vi "Get ICM Setting.vi"(8 "error in (no error)":errorcluster, 10 "Scan Data Process in":T1, 11 "tdms file":refnum<k34>) -> (0 "error out":errorcluster, 2 "Scan Data Process out":T1, 3 "tdms file out":refnum<k34>, 4 "Vaild?":bool)   [LabVIEW 2015, in "Exposure Process.lvlib"]
uses:
  Exposure Process.lvlib
  Control_Scan Data Process.ctl
  <vilib>/addons/PointValueMap/controls/PointMap.ctl
  Control_EXP Information.ctl
  Control_File Save Setup.ctl
  Control_Enable and Path.ctl
  Control_ICM Export Setting.ctl
  <vilib>/addons/PointValueMap/PointValueMap.lvlib
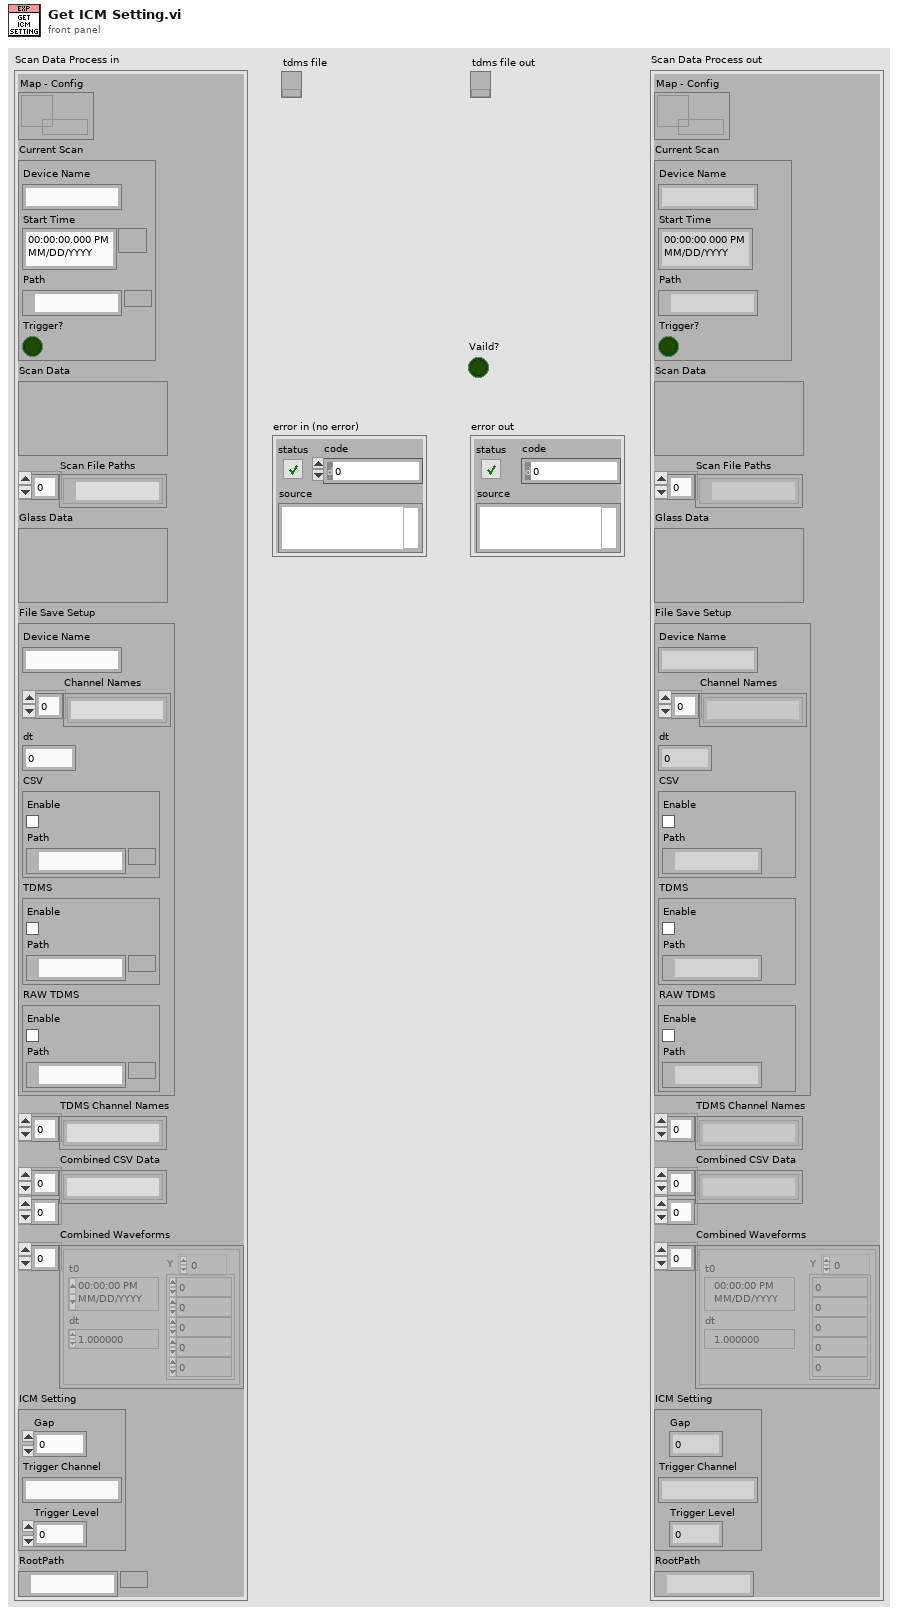
[diagram p1: front panel]
types:
  T1 = typedef "Exposure Process.lvlib/Control_Scan Data Process.ctl" = cluster{"Map - Config":T2, "Current Scan":T3, "Scan Data":variant, "Scan File Paths":path[], "Glass Data":variant, "File Save Setup":T4, "TDMS Channel Names":string[], "Combined CSV Data":string[][], "Combined Waveforms":waveform(dbl)[], "ICM Setting":T6, "RootPath":path}
  T2 = typedef "PointValueMap.lvlib/PointMap.ctl" = refnum<data-value>
  T3 = typedef "Exposure Process.lvlib/Control_EXP Information.ctl" = cluster{"Device Name":string, "Start Time":timestamp, "Path":path, "Trigger?":bool}
  T4 = typedef "Exposure Process.lvlib/Control_File Save Setup.ctl" = cluster{"Device Name":string, "Channel Names":string[], "dt":dbl, "CSV":T5, "TDMS":T5, "RAW TDMS":T5}
  T5 = typedef "Exposure Process.lvlib/Control_Enable and Path.ctl" = cluster{"Enable":bool, "Path":path}
  T6 = typedef "Exposure Process.lvlib/Control_ICM Export Setting.ctl" = cluster{"Gap":dbl, "Trigger Channel":string, "Trigger Level":dbl}
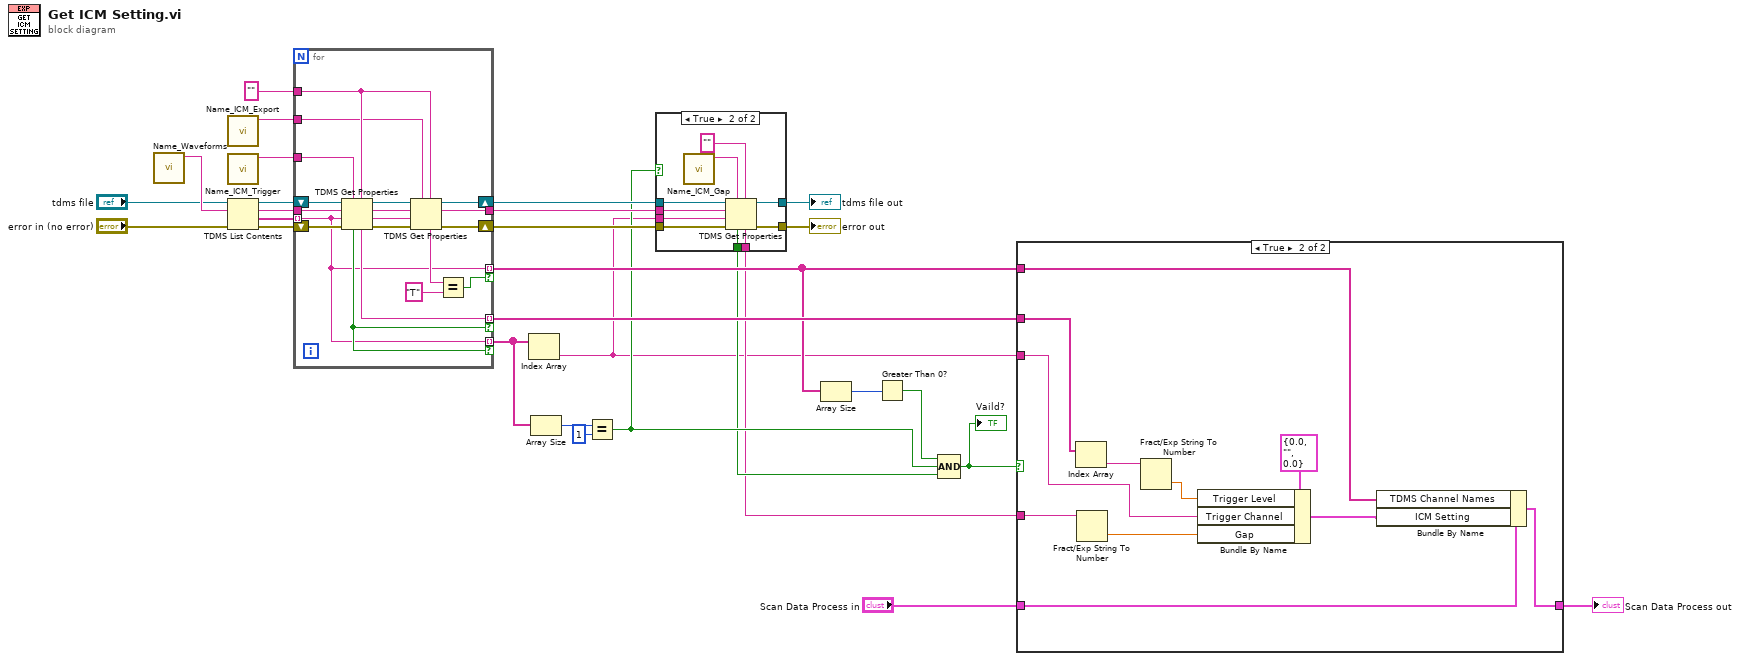
[diagram p0: block diagram]
diagram:
  n1 = call "Name_Waveforms.vi"() -> ("Name"=w13:string)  [unwired: 11 in]
  n2 = call "Name_ICM_Export.vi"() -> ("Name"=w22:string)  [unwired: 11 in]
  n3 = call "Name_ICM_Trigger.vi"() -> ("Name"=w25:string)  [unwired: 11 in]
  n4 = TDMS List Contents(4:"error in (no error)", 6:w13, 7:"tdms file") -> (0:w26:errorcluster, 1:w27:string[], 2:w28:string, 3:w29:refnum<k34>)
  n5 = for {
    tunnel: w28 -> [w46]
    tunnel: w27 -> [w31] mode=indexing
    shift-right: [w40] -> w12
    shift-left: w29 -> [w48]
    shift-right: [w39] -> w11
    shift-left: w26 -> [w47]
    tunnel: w25 -> [w45]
    tunnel: "" -> [w36]
    tunnel: [w44] -> w23 mode=indexing if=w43
    tunnel: [w31] -> w2 mode=indexing if=w43
    tunnel: w22 -> [w35]
    tunnel: [w31] -> w14 mode=indexing if=w32
    tunnel: [w30] -> w10
    n6 = TDMS Get Properties(5:w36, 7:w45, 8:w47, 9:w31, 10:w46, 11:w48) -> (0:w41:errorcluster, 1:w37:string, 2:w38:string, 3:w42:refnum<k34>, 4:w44:string, 6:w43:bool)
    n7 = TDMS Get Properties(5:w36, 7:w35, 8:w41, 9:w37, 10:w38, 11:w42) -> (0:w39:errorcluster, 2:w30:string, 3:w40:refnum<k34>, 4:w33:string)  [unwired: 2 out]
    n8 = Equal?(x=w33, y="T") -> (x = y?=w32:bool)
  }
  n9 = Index Array(array=w2) -> (element=w1:string)  [unwired: 1 in]
  n10 = Array Size(array=w2) -> (size(s)=w20:i32)
  n11 = Equal?(x=w20, y=1) -> (x = y?=w7:bool)
  n12 = case shown="True" w7 {
    tunnel: w12 -> [w50 w58]
    tunnel: w11 -> [w49 w57]
    tunnel: w10 -> [_ w56]
    tunnel: [w50 w55] -> w9
    tunnel: [w49 w54] -> w8
    tunnel: [_ w53] -> w6
    tunnel: [_ w52] -> w5
    tunnel: w1 -> [_ w51]
    frame False {
    }
    frame True {
      n13 = call "Name_ICM_Gap.vi"() -> ("Name"=w60:string)  [unwired: 11 in]
      n14 = TDMS Get Properties(5:"", 7:w60, 8:w57, 9:w51, 10:w56, 11:w58) -> (0:w54:errorcluster, 3:w55:refnum<k34>, 4:w52:string, 6:w53:bool)  [unwired: 2 out]
    }
  }
  "tdms file out" <- w9
  "error out" <- w8
  n15 = Array Size(array=w14) -> (size(s)=w21:i32)
  n16 = Greater Than 0?(x=w21) -> (x > 0?=w18:bool)
  n17 = Compound Arithmetic op=AND(w18, w7, w6) -> (w15:bool)
  "Vaild?" <- w15
  n18 = case shown="True" w15 {
    tunnel: w5 -> [_ w70]
    tunnel: w23 -> [_ w69]
    tunnel: "Scan Data Process in" -> [w61 w65]
    tunnel: [w61 w64] -> w16
    tunnel: w14 -> [_ w63]
    tunnel: w1 -> [_ w62]
    frame False {
    }
    frame True {
      n19 = Index Array(array=w69) -> (element=w68:string)  [unwired: 1 in]
      n20 = Fract/Exp String To Number(string=w70) -> (number=w71:dbl)  [unwired: 3 in, 1 out]
      n21 = Fract/Exp String To Number(string=w68) -> (number=w67:dbl)  [unwired: 3 in, 1 out]
      n22 = Bundle By Name(cluster=T6 {"Gap"=0.0, "Trigger Channel"="", "Trigger Level"=0.0} ("ICM Setting"), "Trigger Level"=w67, "Trigger Channel"=w62, "Gap"=w71) -> (w66:T6)
      n23 = Bundle By Name(cluster=w65, "TDMS Channel Names"=w63, "ICM Setting"=w66) -> (w64:T1)
    }
  }
  "Scan Data Process out" <- w16
